vi "ScaleTraj_Height.vi"(8 "Enum":enum16{"3D", "2D"}(ring)=enum."2D", 10 "ScalingCoef":dbl=1.0, 11 "Averaged Gait":dbl[][](array[numeric])) -> (2 "ScaledGait":dbl[][](array[numeric]), 3 "XY Graph":cluster{"Y":dbl[], "Y":dbl[]}[](graph))   [LabVIEW 2016]
uses:
  <userlib>/_OpenG.lib/array/array.llb/Index 1D Array Elements (DBL)__ogtk.vi
  <vilib>/imath/engines/lvmath2/RunTimeEngine/IndexRead/NIMS V(S).vi
  <instcachedir>/0/NIMS V(S)_0488751826AF41519A22953C041130DC.lvgen/NIMS V(S)_0488751826AF41519A22953C041130DC_000.vi
  <vilib>/imathl/engines/lvmath/Functions/Error Handling/Create Error.vi
  <vilib>/imath/engines/lvmath2/RunTimeEngine/ArithmeticOperatorToken/NIMS_ArithmeticOperator_power(S).vi
  <instcachedir>/0/NIMS_ArithmeticOperator_power(S)_1E6AB98FD36540B9B758A69A385A1B47.lvgen/NIMS_ArithmeticOperator_power(S)_1E6AB98FD36540B9B758A69A385A1B47_015.vi
  <instcachedir>/0/NIMS_ArithmeticOperator_power(S)_1E6AB98FD36540B9B758A69A385A1B47.lvgen/NIMS_ArithmeticOperator_power(S)_1E6AB98FD36540B9B758A69A385A1B47_014.vi
  <vilib>/imath/engines/lvmath2/RunTimeEngine/ErrorHandling/NIMS_Create Error From Enums.vi
  <vilib>/imath/engines/lvmath2/RunTimeEngine/NodeEndStatement/NIMS_NodeEndStatement_Output.vi
  <instcachedir>/0/NIMS_NodeEndStatement_Output_53EC0D466D134D7ABD903AC30B43404B.lvgen/NIMS_NodeEndStatement_Output_53EC0D466D134D7ABD903AC30B43404B_005.vi
  <vilib>/imath/engines/lvmath2/RunTimeEngine/ErrorHandling/NIMS_Finalize Error.vi
panel:
  out "XY Graph 2":cluster{dbl[], "yi":dbl[]}(graph)
  out "XY":cluster{"Mean":dbl[], "Mean":dbl[]}[](array[cluster])
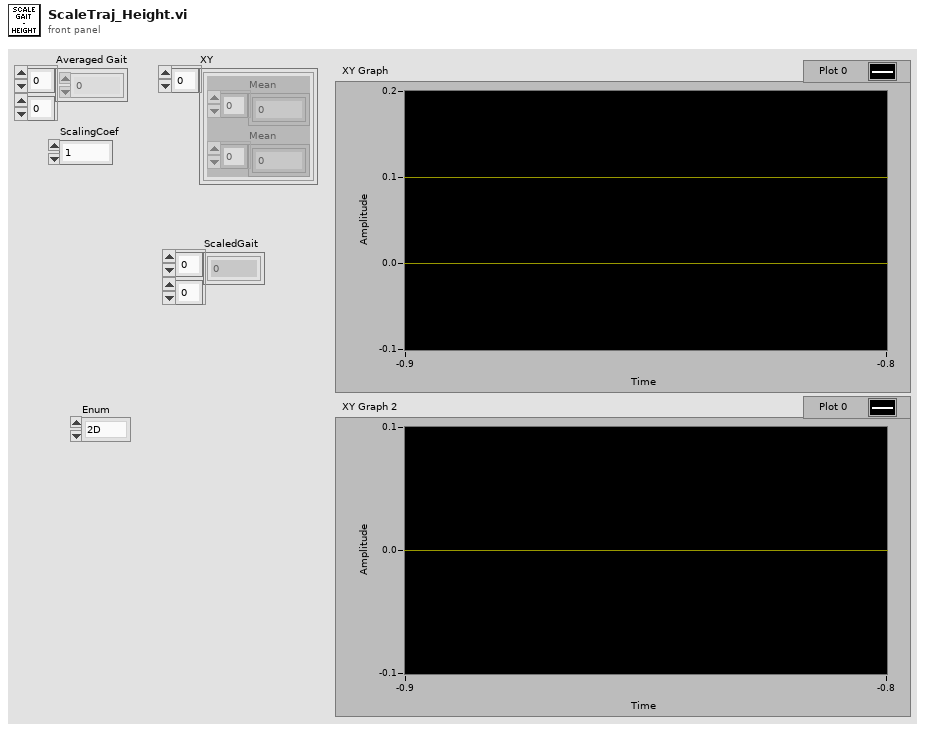
[diagram p1: front panel]
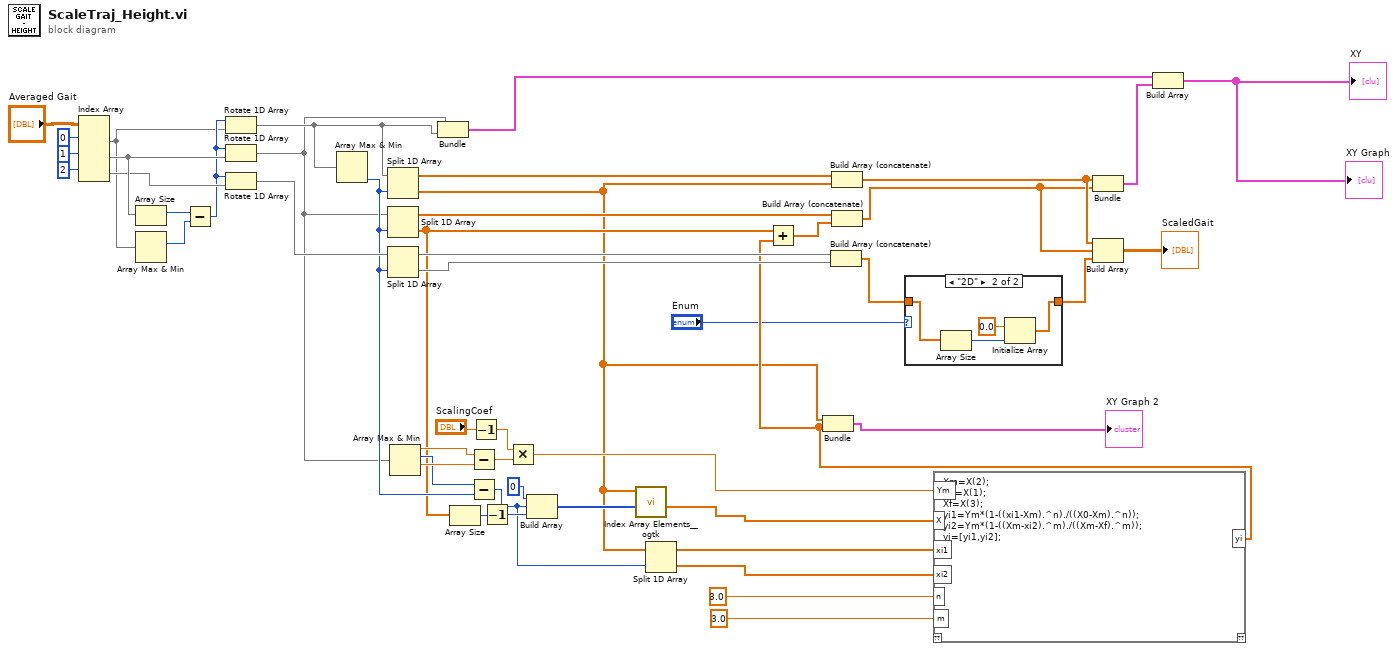
[diagram p0: block diagram]
diagram:
  n1 = Index Array(array="Averaged Gait", index (row) #1=0 ("index (row)"), index (row) #2=1 ("index (row)"), index (row) #3=2 ("index (row)")) -> (element #1=w37:dbl[], element #2=w45:dbl[], element #3=w41:dbl[])  [unwired: 3 in]
  n2 = Array Size(array=w45) -> (size(s)=w44:i32)
  n3 = Array Max & Min(array=w37) -> (max index (indices)=w43:i32)  [unwired: 3 out]
  n4 = Subtract(x=w44, y=w43) -> (x-y=w40:i32)
  n5 = Rotate 1D Array(1:w37, 2:w40) -> (0:w4:dbl[])
  n6 = Rotate 1D Array(1:w45, 2:w40) -> (0:w3:dbl[])
  n7 = Rotate 1D Array(1:w41, 2:w40) -> (0:w38:dbl[])
  n8 = Array Max & Min(array=w4) -> (min index (indices)=w24:i32)  [unwired: 3 out]
  n9 = Split 1D Array(array=w4, index=w24) -> (first subarray=w30:dbl[], second subarray=w13:dbl[])
  n10 = Split 1D Array(array=w3, index=w24) -> (first subarray=w31:dbl[], second subarray=w20:dbl[])
  n11 = Split 1D Array(array=w38, index=w24) -> (first subarray=w29:dbl[], second subarray=w28:dbl[])
  n12 = Array Max & Min(array=w3) -> (max value=w33:dbl, max index (indices)=w25:i32, min value=w34:dbl)  [unwired: 1 out]
  n13 = Bundle(w3, w4) -> (w49:cluster{dbl[], dbl[]})  [unwired: 1 in]
  n14 = Array Size(array=w20) -> (size(s)=w36:i32)
  n15 = Subtract(x=w33, y=w34) -> (x-y=w22:dbl)
  n16 = Subtract(x=w25, y=w24) -> (x-y=w12:i32)
  n17 = Decrement(x="ScalingCoef") -> (x-1=w21:dbl)
  n18 = Decrement(x=w36) -> (x-1=w23:i32)
  n19 = Multiply(x=w21, y=w22) -> (x*y=w17:dbl)
  n20 = Build Array(0 ("element"), w12, w23) -> (w18:i32[])
  n21 = call-poly <userlib>:"Index Array Elements__ogtk.vi"("indices"=w18, "array"=w13) -> ("elements"=w16:dbl[])  [unwired: 9 in]
  n22 = Split 1D Array(array=w13, index=w12) -> (first subarray=w11:dbl[], second subarray=w10:dbl[])
  n23 = Build Array (concatenate)(w29, w28) -> (w6:dbl[])
  n24 = Build Array (concatenate)(w30, w13) -> (w2:dbl[])
  n25 = case shown="\"2D\"" "Enum" {
    tunnel: w6 -> [w50 w54]
    tunnel: [w50 w52] -> w5
    frame "3D", Default {
    }
    frame "2D" {
      n26 = Array Size(array=w54) -> (size(s)=w53:i32)
      n27 = Initialize Array(0.0 ("element"), w53) -> (w52:dbl[])
    }
  }
  n28 = mathscript code="Xm=X(2);\nX0=X(1);\nXf=X(3);\nyi1=Ym*(1-((xi1-Xm).^n)./((X0-Xm).^n));\nyi2=Ym*(1-((Xm-xi2).^m)./((Xm-Xf).^m));\nyi=[yi1,yi2];"("Ym"=w17, "X"=w16, "xi1"=w11, "n"=3.0 ("element"), "xi2"=w10, "m"=3.0 ("element")) -> ("yi"=w14:dbl[])  [unwired: 1 in, 1 out]
  n29 = Add(x=w20, y=w14) -> (x+y=w32:dbl[])
  n30 = Bundle(w13, "yi"=w14) -> (→"XY Graph 2":cluster{dbl[], "yi":dbl[]})  [unwired: 1 in]
  n31 = Build Array (concatenate)(w31, w32) -> (w1:dbl[])
  n32 = Bundle(w2, w1) -> (w27:cluster{dbl[], dbl[]})  [unwired: 1 in]
  n33 = Build Array(w2, w1, w5) -> (→"ScaledGait":dbl[][])
  n34 = Build Array(w49, w27) -> (→"XY" →"XY Graph":cluster{dbl[], dbl[]}[])
